vi "Stop Task.vi"(8 "error in":errorcluster, 11 "NI Waveform Output in":refnum<class "NI Waveform Output.lvclass">) -> (0 "error out":errorcluster, 3 "NI Waveform Output out":refnum<class "NI Waveform Output.lvclass">)   [LabVIEW 2023, in "HardwareAbstractionLayer_LVOOP.lvlib" / "NI Waveform Output.lvclass"]
doc: "This VI is DAQmx Stop the Task"
uses:
  NI Waveform Output.lvclass
  NI Waveform Output.lvclass/NI Waveform Output.ctl
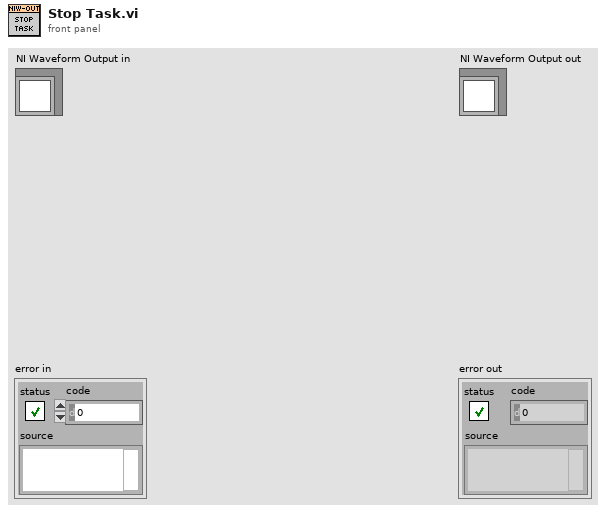
[diagram p1: front panel]
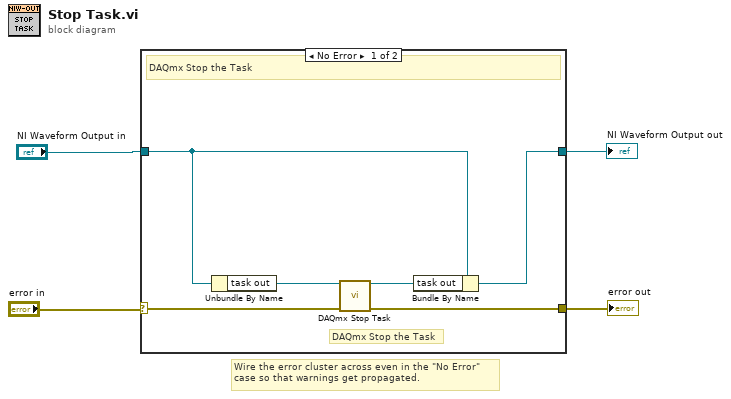
[diagram p0: block diagram]
diagram:
  # "Wire the error cluster across even in the \"No Error\"\ncase so that warnings get propagated."
  n1 = case shown="No Error" "error in" {
    selector: "error in" -> [w10 w12]
    tunnel: [w9 w12] -> w3
    tunnel: [w6 w11] -> w1
    tunnel: "NI Waveform Output in" -> [w7 w11]
    frame No Error {
      # "DAQmx Stop the Task"
      # "DAQmx Stop the Task"
      n2 = Unbundle By Name(w7) -> ("task out"=w8:refnum<k21>)
      n3 = call <vilib>:"DAQmx Stop Task.vi"("task/channels in"=w8, "error in"=w10) -> ("task out"=w5:refnum<k21>, "error out"=w9:errorcluster)  [unwired: 12 in]
      n4 = Bundle By Name(cluster=w7, "task out"=w5) -> (w6:refnum<class "NI Waveform Output.lvclass">)
    }
    frame Error {
    }
  }
  "error out" <- w3
  "NI Waveform Output out" <- w1
